vi "WriteHwStatusToMap.vi"(8 "error in (no error)":errorcluster, 10 "Map in":T11, 11 "Group":T1) -> (0 "error out":errorcluster, 2 "Map out":T11, 3 "Group out":T1)   [LabVIEW 2017, in "McsaAnalysisLowRate.lvlib"]
uses:
  <vilib>/addons/InsightCM/Devices/Shared/Mcsa/McsaAnalysisLowRate/McsaAnalysisLowRate.lvlib
  <vilib>/addons/PointValueMap/PointValueMap.lvlib
  <vilib>/addons/PointValueMap/controls/PointMap.ctl
  <vilib>/addons/InsightCM/Utilities/Analysis/Shared/controls/Feature.ctl
  <vilib>/addons/InsightCM/Utilities/Analysis/Shared/AnalysisHelper.lvlib
  <vilib>/addons/InsightCM/Utilities/Analysis/Shared/controls/AmplitudeScale.ctl
  <vilib>/addons/InsightCM/Utilities/Analysis/MCSA/controls/McsaChannelPhasor.ctl
  <vilib>/addons/InsightCM/Utilities/Analysis/MCSA/McsaAnalysisFunctions.lvlib
  <vilib>/addons/InsightCM/Devices/Shared/Mcsa/McsaAnalysisLowRate/controls/Group.ctl
  <vilib>/addons/InsightCM/MessageBus/Base/controls/KeyValuePair.ctl
  <vilib>/addons/Electrical Power/Basic/Measurement/subVIs/basic_Power Value.ctl
  <vilib>/addons/Electrical Power/Basic/NI_EP_Basic.lvlib
  <vilib>/addons/InsightCM/Utilities/Analysis/MCSA/controls/TorqueLoadEfficiency.ctl
  <vilib>/addons/InsightCM/Utilities/Analysis/MCSA/controls/MotorCalculationCache.ctl
  <vilib>/addons/InsightCM/Utilities/Analysis/MCSA/controls/McsaChannel.ctl
  <vilib>/addons/InsightCM/Utilities/Analysis/MCSA/controls/McsaMotor.ctl
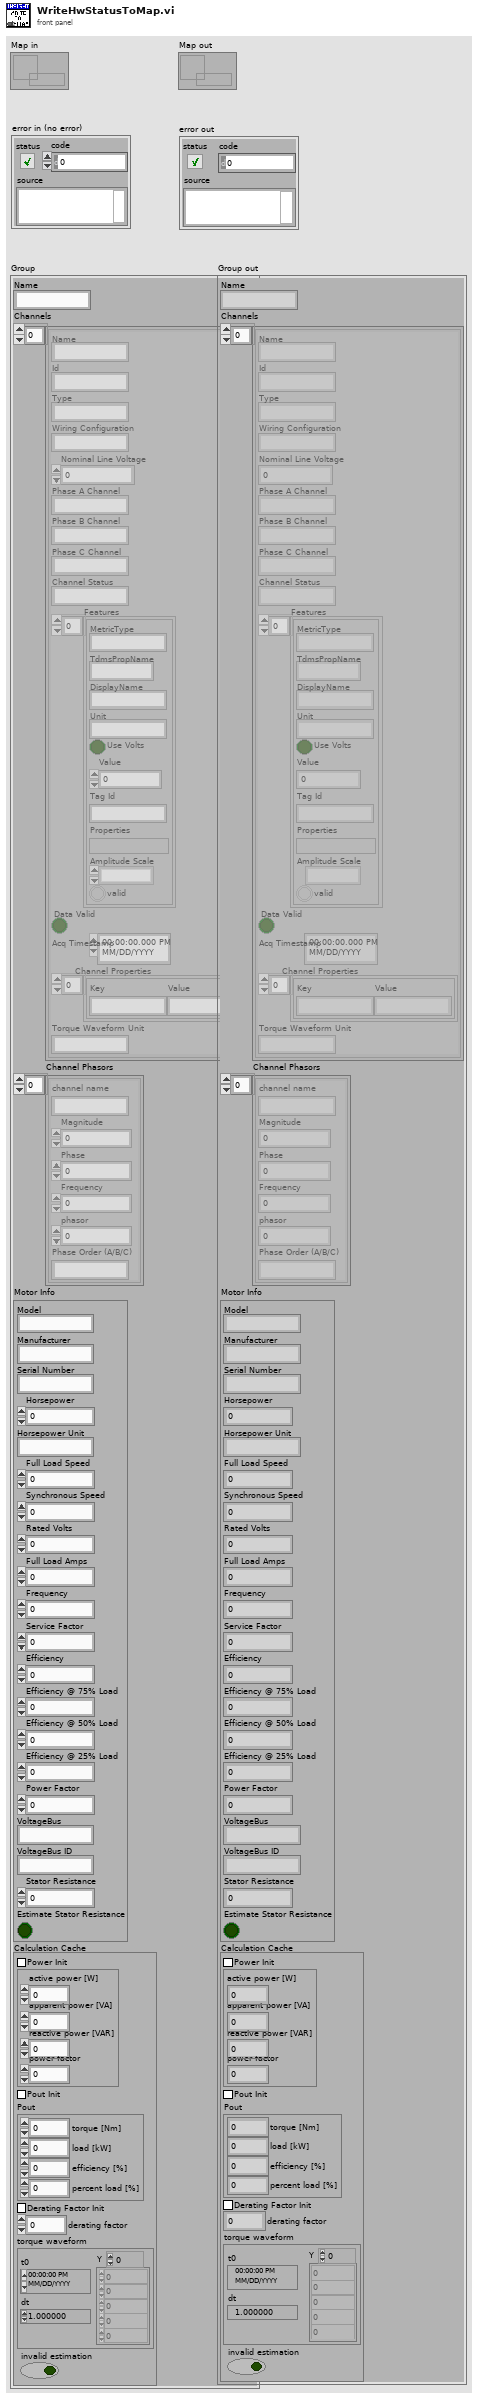
[diagram p1: front panel]
types:
  T1 = typedef "McsaAnalysisLowRate.lvlib/Group.ctl" = cluster{"Name":string, "Channels":T2[], "Channel Phasors":T6[], "Motor Info":T7, "Calculation Cache":T8}
  T2 = typedef "McsaAnalysisFunctions.lvlib/McsaChannel.ctl" = cluster{"Name":string, "Id":string, "Type":string, "Wiring Configuration":string, "Nominal Line Voltage":dbl, "Phase A Channel":string, "Phase B Channel":string, "Phase C Channel":string, "Channel Status":string, "Features":T3[], "Data Valid":bool, "Acq Timestamp":timestamp, "Channel Properties":T5[], "Torque Waveform Unit":string}
  T3 = typedef "AnalysisHelper.lvlib/Feature.ctl" = cluster{"MetricType":string, "TdmsPropName":string, "DisplayName":string, "Unit":string, "Use Volts":bool, "Value":dbl, "Tag Id":string, "Properties":variant, "Amplitude Scale":T4, "valid":bool}
  T4 = typedef "AnalysisHelper.lvlib/AmplitudeScale.ctl" = enum16{"rms", "peak", "pk-pk"}
  T5 = typedef "KeyValuePair.ctl" = cluster{"Key":string, "Value":string}
  T6 = typedef "McsaAnalysisFunctions.lvlib/McsaChannelPhasor.ctl" = cluster{"channel name":string, "Magnitude":dbl, "Phase":dbl, "Frequency":dbl, "phasor":cdb, "Phase Order (A/B/C)":string}
  T7 = typedef "McsaAnalysisFunctions.lvlib/McsaMotor.ctl" = cluster{"Model":string, "Manufacturer":string, "Serial Number":string, "Horsepower":dbl, "Horsepower Unit":string, "Full Load Speed":dbl, "Synchronous Speed":dbl, "Rated Volts":dbl, "Full Load Amps":dbl, "Frequency":dbl, "Service Factor":dbl, "Efficiency":dbl, "Efficiency @ 75% Load":dbl, "Efficiency @ 50% Load":dbl, "Efficiency @ 25% Load":dbl, "Power Factor":dbl, "VoltageBus":string, "VoltageBus ID":string, "Stator Resistance":dbl, "Estimate Stator Resistance":bool}
  T8 = typedef "McsaAnalysisFunctions.lvlib/MotorCalculationCache.ctl" = cluster{"Power Init":bool, "power value":T9, "Pout Init":bool, "Pout":T10, "Derating Factor Init":bool, "derating factor":sgl, "torque waveform":waveform(dbl), "invalid estimation":bool}
  T9 = typedef "NI_EP_Basic.lvlib/basic_Power Value.ctl" = cluster{"active power [W]":dbl, "apparent power [VA]":dbl, "reactive power [VAR]":dbl, "power factor":dbl}
  T10 = typedef "McsaAnalysisFunctions.lvlib/TorqueLoadEfficiency.ctl" = cluster{"torque [Nm]":dbl, "load [kW]":dbl, "efficiency [%]":dbl, "percent load [%]":dbl}
  T11 = typedef "PointValueMap.lvlib/PointMap.ctl" = refnum<data-value>
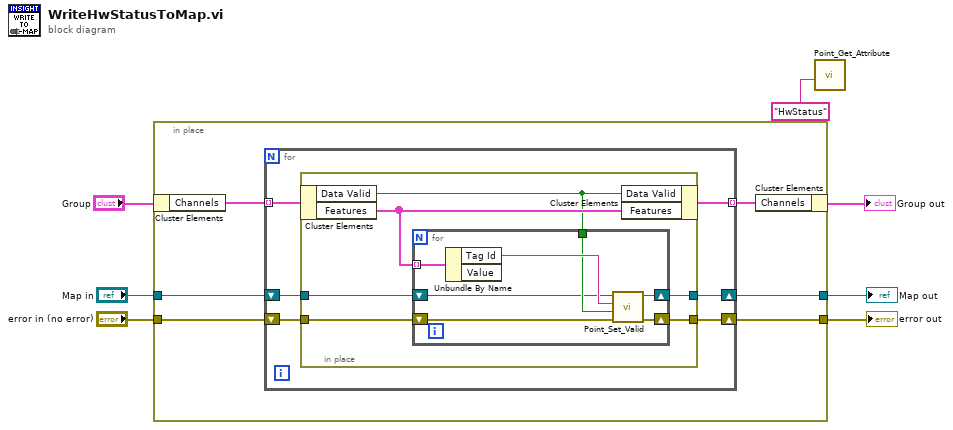
[diagram p0: block diagram]
diagram:
  n1 = in-place {
    in-place-border: "Map in" -> [w9]
    in-place-border: "error in (no error)" -> [w8]
    in-place-border: [w10] -> w7
    in-place-border: [w13] -> w4
    n2 = in-place-cluster #1("Group") -> ("Channels"=w12:T2[])
    n3 = for {
      tunnel: w12 -> [w19] mode=indexing
      shift-right: [w15] -> w13
      shift-left: w9 -> [w18]
      tunnel: [w14] -> w11 mode=indexing
      shift-right: [w16] -> w10
      shift-left: w8 -> [w17]
      n4 = in-place {
        in-place-border: w18 -> [w25]
        in-place-border: w17 -> [w24]
        in-place-border: [w21] -> w16
        in-place-border: [w23] -> w15
        n5 = in-place-cluster #2(w19) -> ("Data Valid"=w20:bool, "Features"=w22:T3[])
        n6 = for {
          tunnel: w22 -> [w32] mode=indexing
          shift-right: [w31] -> w23
          shift-left: w25 -> [w27]
          shift-right: [w30] -> w21
          shift-left: w24 -> [w26]
          tunnel: w20 -> [w28]
          n7 = Unbundle By Name(w32) -> ("Tag Id"=w29:string)  [unwired: 1 out]
          n8 = call <vilib>:"Point_Set_Valid.vi"("Error In"=w26, "Valid?"=w28, "Tag"=w29, "Map"=w27) -> ("Error Out"=w30:errorcluster, "Map Out"=w31:T11)  [unwired: 6 in]
        }
        n9 = in-place-cluster #2("Data Valid"=w20, "Features"=w22) -> (w14:T2)
      }
    }
    n10 = in-place-cluster #1("Channels"=w11) -> (→"Group out":T1)
  }
  "error out" <- w7
  "Map out" <- w4
  n11 = call <vilib>:"Point_Get_Attribute.vi"("Attribute"="HwStatus") -> ()  [unwired: 7 in, 4 out]
